vi "Identity Matrix.vi"(1 "matrix size":i32=4) -> (0 "Identity Matrix":T1)   [LabVIEW 2024]
uses:
  <vilib>/Analysis/7linalg.llb/Create Special Real Matrix.vi
  <vilib>/Analysis/NI_AALPro.lvlib
  <vilib>/Analysis/Matrix/Datatypes/RealMatrix.ctl
  <vilib>/Analysis/Matrix/NI_Matrix.lvlib
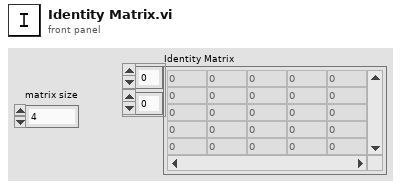
[diagram p1: front panel]
types:
  T1 = typedef "NI_Matrix.lvlib/RealMatrix.ctl" = dbl[][]
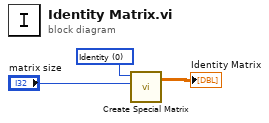
[diagram p0: block diagram]
diagram:
  w3 = 0 items=["Identity", "Diagonal", "Toeplitz", "Vandermonde", "Companion", "Hankel", "Hadamard", "Wilkinson", "Hilbert", "Inverse Hilbert", "Rosser", "Pascal"] ("matrix type")
  n1 = call-poly <vilib>:"Create Special Matrix.vi"("matrix type"=w3, "matrix size"="matrix size") -> ("Special Matrix"=→"Identity Matrix":T1)  [unwired: 3 in, 1 out]
